vi "Initialize.vi"(8 "error in (no error)":errorcluster, 11 "VictorDrive in":refnum<class "VictorDrive.lvclass">) -> (0 "error out":errorcluster, 3 "VictorDrive out":refnum<class "VictorDrive.lvclass">)   [LabVIEW 2017, in "Drive.lvlib" / "VictorDrive.lvclass"]
uses:
  VictorDrive.lvclass
  <vilib>/Rock Robotics/SystemInterfaces/DIO/FPGA_DIOPWMChannel.ctl
  <vilib>/Rock Robotics/WPI/SafetyOutput/WPI_SafetyOutputConfigMenu.ctl
  VictorDrive.lvclass/VictorDrive.ctl
  <vilib>/Rock Robotics/WPI/MotorControl/WPI_MotorControlOpen Victor.vi
  <vilib>/Rock Robotics/WPI/RobotDrive/WPI_RobotDriveOpen4MotorWithExistingMotors.vi
  Drive.lvclass
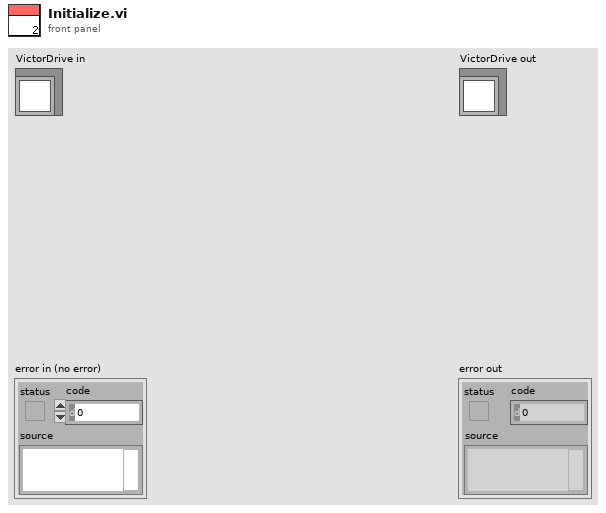
[diagram p1: front panel]
types:
  T1 = typedef "WPI_SafetyOutputConfigMenu.ctl" = enum16{"Enable", "Disable"}
  T2 = typedef "FPGA_DIOPWMChannel.ctl" = enum8{"PWM 0", "PWM 1", "PWM 2", "PWM 3", "PWM 4", "PWM 5", "PWM 6", "PWM 7", "PWM 8", "PWM 9", "PWM MXP 0", "PWM MXP 1", "PWM MXP 2", "PWM MXP 3", "PWM MXP 4", "PWM MXP 5", "PWM MXP 6", "PWM MXP 7", "PWM MXP 8", "PWM MXP 9", "Invalid"}
  T3 = typedef "WPI_MotorControlDeviceRef.ctl" = cluster{"DeviceStatus":errorcluster, "Type":T4, "PWM":cluster{"PWM Channel":T2, "DeadBand":T5}, "CAN":cluster{"Device Number":u8, "SetOutput VI Ref":variant, "GetOutput VI Ref":variant, "Enable VI Ref":variant, "Disable VI Ref":variant, "Data":variant}, "Invert":bool, "DIO PWM":cluster{"PWM \"Enable\" Channel":T2, "DIOChannel":T6, "PWM Rate":dbl}}
  T4 = typedef "WPI_MotorControlType.ctl" = enum16{"PWM", "CAN", "DIO PWM"}
  T5 = typedef "WPI_PWMDeadband.ctl" = cluster{"Name":string, "maxPositivePwm":i32, "minPositivePwm":i32, "centerPwm":i32, "maxNegativePwm":i32, "minNegativePwm":i32, "angularRange":u16}
  T6 = typedef "FPGA_DIOChannel.ctl" = enum8{"DIO 0", "DIO 1", "DIO 2", "DIO 3", "DIO 4", "DIO 5", "DIO 6", "DIO 7", "DIO 8", "DIO 9", "DIO MXP 0", "DIO MXP 1", "DIO MXP 2", "DIO MXP 3", "DIO MXP 4", "DIO MXP 5", "DIO MXP 6", "DIO MXP 7", "DIO MXP 8", "DIO MXP 9", "DIO MXP 10", "DIO MXP 11", "DIO MXP 12", "DIO MXP 13", "DIO MXP 14", "DIO MXP 15", "SPI Port CS1", "SPI Port CS2", "SPI Port CS3", "SPI Port MISO", "SPI Port MOSI", "Invalid"}
  T7 = typedef "WPI_RobotDriveDevRef.ctl" = cluster{"DevStatus":errorcluster, "Motors[]":T3[], "Square Inputs":bool, "Max Output":dbl}
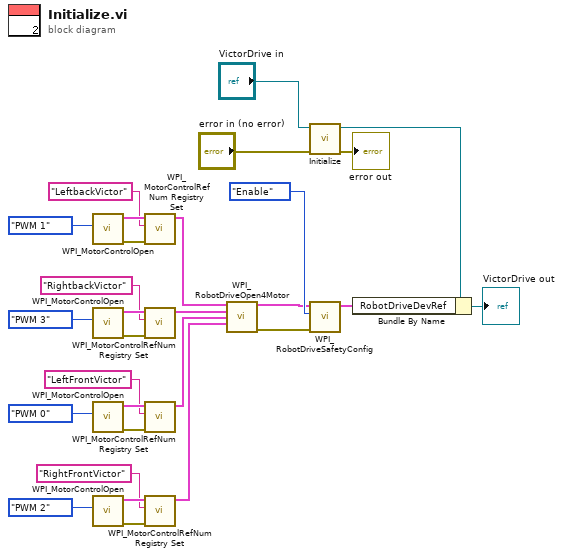
[diagram p0: block diagram]
diagram:
  n1 = call-poly <vilib>:"WPI_MotorControlOpen.vi"("PWM Channel"=FPGA_DIOPWMChannel."PWM 1") -> ("error out"=w25:errorcluster, "MotorControlDeviceRef"=w26:T3)  [unwired: 9 in]
  n2 = call-poly <vilib>:"WPI_MotorControlOpen.vi"("PWM Channel"=FPGA_DIOPWMChannel."PWM 3") -> ("error out"=w21:errorcluster, "MotorControlDeviceRef"=w22:T3)  [unwired: 9 in]
  n3 = call-poly <vilib>:"WPI_MotorControlOpen.vi"("PWM Channel"=FPGA_DIOPWMChannel."PWM 0") -> ("error out"=w17:errorcluster, "MotorControlDeviceRef"=w18:T3)  [unwired: 9 in]
  n4 = call-poly <vilib>:"WPI_MotorControlOpen.vi"("PWM Channel"=FPGA_DIOPWMChannel."PWM 2") -> ("error out"=w13:errorcluster, "MotorControlDeviceRef"=w14:T3)  [unwired: 9 in]
  n5 = call <vilib>:"WPI_MotorControlRefNum Registry Set.vi"("error in (no error)"=w25, "refnum name"="LeftbackVictor", "MotorControlDevRef"=w26) -> ("MotorControlDevRef"=w7:T3)  [unwired: 7 in, 1 out]
  n6 = call <vilib>:"WPI_MotorControlRefNum Registry Set.vi"("error in (no error)"=w21, "refnum name"="RightbackVictor", "MotorControlDevRef"=w22) -> ("MotorControlDevRef"=w8:T3)  [unwired: 7 in, 1 out]
  n7 = call <vilib>:"WPI_MotorControlRefNum Registry Set.vi"("error in (no error)"=w17, "refnum name"="LeftFrontVictor", "MotorControlDevRef"=w18) -> ("MotorControlDevRef"=w9:T3)  [unwired: 7 in, 1 out]
  n8 = call <vilib>:"WPI_MotorControlRefNum Registry Set.vi"("error in (no error)"=w13, "refnum name"="RightFrontVictor", "MotorControlDevRef"=w14) -> ("MotorControlDevRef"=w10:T3)  [unwired: 7 in, 1 out]
  n9 = call-poly <vilib>:"WPI_RobotDriveOpen4Motor.vi"("Rear Left Motor Dev Ref"=w7, "Rear Right Motor Dev Ref"=w8, "Front Left Motor Dev Ref"=w9, "Front Right Motor Dev Ref"=w10) -> ("RobotDriveDevRef"=w5:T7, "error out"=w4:errorcluster)  [unwired: 10 in]
  n10 = call-parent "Initialize.vi"("error in (no error)"="error in (no error)", "Drive in"="VictorDrive in") -> ("error out"=→"error out":errorcluster, "Drive out"=w2:refnum<class "VictorDrive.lvclass">)  [unwired: 8 in]
  n11 = call <vilib>:"WPI_RobotDriveSafetyConfig.vi"("error in (no error)"=w4, "mode"=WPI_SafetyOutputConfigMenu."Enable", "RobotDriveDevRef"=w5) -> ("RobotDriveDevRef"=w3:T7)  [unwired: 7 in, 1 out]
  n12 = Bundle By Name(cluster=w2, "RobotDriveDevRef"=w3) -> (→"VictorDrive out":refnum<class "VictorDrive.lvclass">)
